vi "Sequencer Do.vi"(8 "error in (no error)":errorcluster, 10 "Sequencer in":refnum<class "Sequencer.lvclass">, 11 "Sequencer Msg":refnum<class "Sequencer Msg.lvclass">) -> (0 "error out":errorcluster, 2 "Sequencer out":refnum<class "Sequencer.lvclass">)   [LabVIEW 2020, in "Sequencer.lvlib" / "Sequencer Msg.lvclass"]
doc: "The action the Sequencer Msg performs in the Sequencers Recieve Message method.\nThe default implementation forwards the message to hte Sequencer Core."
uses:
  Sequencer Msg.lvclass
  C:/Current projects/WS/PPL/HDH.Actor Framework.Core.Actor.lvlibp/1abvi3w/vi.lib/ActorFramework/Message/Message.lvclass
  Sequencer/Sequencer.lvclass
  Sequencer Msg.lvclass/Sequencer Msg.ctl
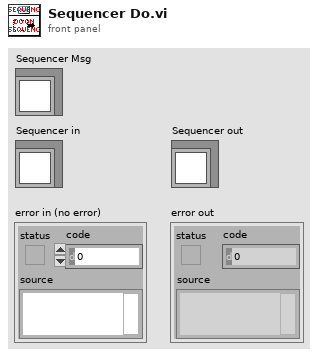
[diagram p1: front panel]
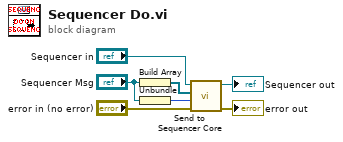
[diagram p0: block diagram]
diagram:
  n1 = Build Array("Sequencer Msg") -> (w1:refnum<class "Sequencer Msg.lvclass">[])
  n2 = Unbundle("Sequencer Msg") -> (w5:u16)
  n3 = call "Send to Sequencer Core.vi"("error in (no error)"="error in (no error)", "Message Priority"=w5, "Message Array"=w1, "Sequencer in"="Sequencer in") -> ("error out"=→"error out":errorcluster, "Sequencer out"=→"Sequencer out":refnum<class "Sequencer.lvclass">)  [unwired: 6 in]
